vi "string to response.vi"(11 "command string":string) -> (2 "invalid":bool, 3 "responses":T1)   [LabVIEW 2013, in "DCAF Execution Service.lvlib"]
uses:
  DCAF Execution Service.lvlib
  common reponses to network process.ctl
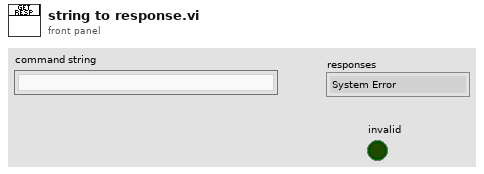
[diagram p1: front panel]
types:
  T1 = typedef "DCAF Execution Service.lvlib/common reponses to network process.ctl" = enum16{"System Error", "Load Report", "Action Response", "Engine Status"}
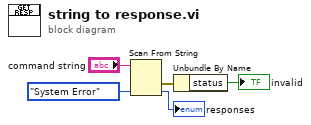
[diagram p0: block diagram]
diagram:
  n1 = Scan From String(input string="command string", default 1=common_reponses_to_network_process."System Error" ("responses")) -> (error out=w4:errorcluster, output 1=→"responses":T1)  [unwired: 3 in, 2 out]
  n2 = Unbundle By Name(w4) -> ("status"=→"invalid":bool)
